vi "TDMS GET DATA G1.vi"(7 "OffSet In":i32, 8 "error in":errorcluster, 10 "max":i64, 11 "tdms file In":refnum<k34>) -> (0 "error out":errorcluster, 3 "Result":cluster{u32, dbl, dbl, dbl, dbl}[](array[cluster]), 4 "lengh":i64, 5 "Repetir":bool)   [LabVIEW 2015]
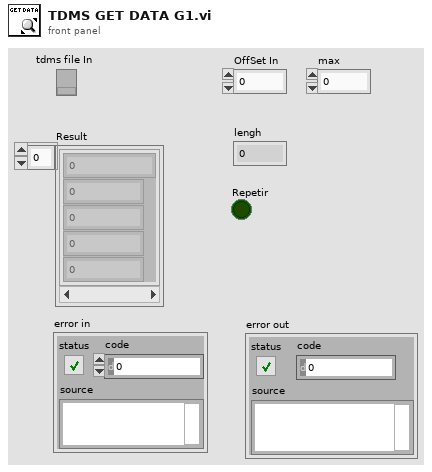
[diagram p1: front panel]
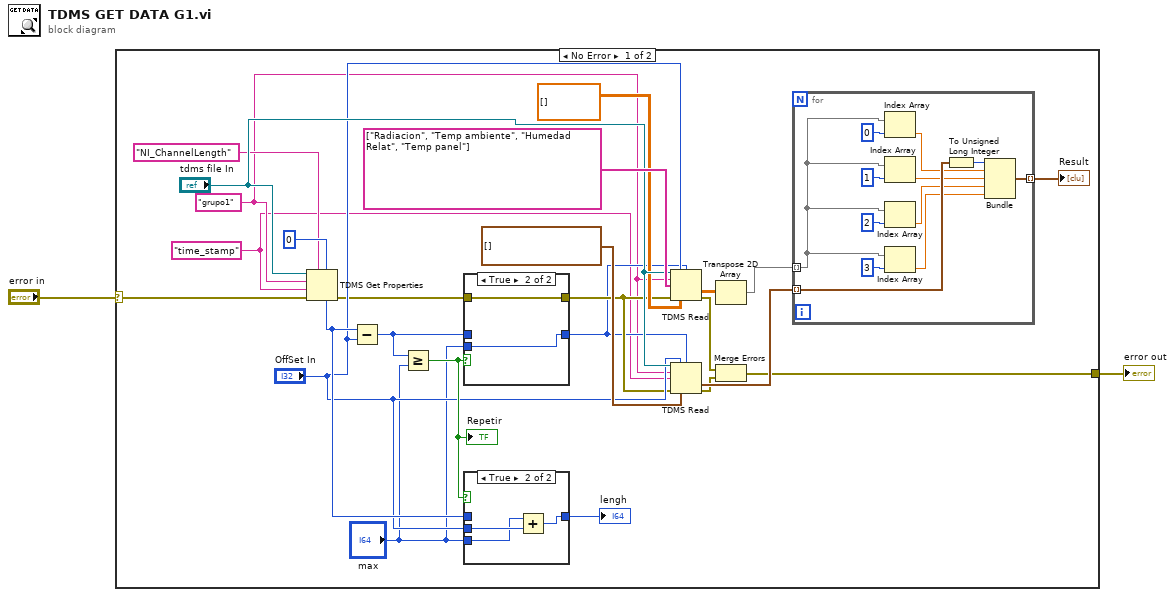
[diagram p0: block diagram]
diagram:
  n1 = case shown="No Error" "error in" {
    selector: "error in" -> [w3 w48]
    tunnel: [w15 w48] -> w2
    frame No Error {
      w6 = "time_stamp"
      w7 = "grupo1"
      n2 = TDMS Get Properties(5:0, 7:"NI_ChannelLength" ("property name"), 8:w3, 9:w6, 10:w7, 11:"tdms file In") -> (0:w11:errorcluster, 4:w13:i32)  [unwired: 4 out]
      n3 = Subtract(x=w13, y="OffSet In") -> (x-y=w18:i32)
      n4 = Greater Or Equal?(x=w18, y="max") -> (x >= y?=w14:bool)
      "Repetir" <- w14
      n5 = case shown="True" w14 {
        tunnel: [w33 w34] -> w8
        tunnel: w18 -> [w33 _]
        tunnel: [w32 w35] -> w9
        tunnel: w11 -> [w32 w35]
        tunnel: "max" -> [_ w34]
        frame False {
        }
        frame True {
        }
      }
      n6 = case shown="True" w14 {
        tunnel: "OffSet In" -> [_ w31]
        tunnel: [w28 w30] -> w4
        tunnel: w13 -> [w28 _]
        tunnel: "max" -> [_ w29]
        frame False {
        }
        frame True {
          n7 = Add(x=w29, y=w31) -> (x+y=w30:i64)
        }
      }
      "lengh" <- w4
      n8 = TDMS Read(0:"tdms file In", 1:"OffSet In", 2:w8, 5:w7, 7:string[] ["Radiacion", "Temp ambiente", "Humedad Relat", "Temp panel"] ("channel name(s) in"), 11:w9, 12:dbl[][] []) -> (10:w24:dbl[][], 15:w17:errorcluster)  [unwired: 1 in, 4 out]
      n9 = TDMS Read(0:"tdms file In", 1:"OffSet In", 2:w8, 5:w7, 7:w6, 11:w9, 12:timestamp[] []) -> (10:w25:timestamp[], 15:w16:errorcluster)  [unwired: 1 in, 4 out]
      n10 = Transpose 2D Array(2D array=w24) -> (transposed array=w23:dbl[][])
      n11 = Merge Errors(w17, w16) -> (w15:errorcluster)
      n12 = for {
        tunnel: w25 -> [w47] mode=indexing
        tunnel: w23 -> [w42] mode=indexing
        tunnel: [w36] -> w22 mode=indexing
        n13 = Index Array(array=w42, index=0) -> (element=w40:dbl)
        n14 = Index Array(array=w42, index=1) -> (element=w39:dbl)
        n15 = Index Array(array=w42, index=2) -> (element=w38:dbl)
        n16 = Index Array(array=w42, index=3) -> (element=w37:dbl)
        n17 = To Unsigned Long Integer(number=w47) -> (unsigned 32bit integer=w41:u32)
        n18 = Bundle(w41, w40, w39, w38, w37) -> (w36:cluster{u32, dbl, dbl, dbl, dbl})  [unwired: 1 in]
      }
      "Result" <- w22
    }
    frame Error {
    }
  }
  "error out" <- w2
